vi "Store Configuration Parameters.vi"(8 "error in (no error)":errorcluster, 10 "refnum":T1, 11 "VacuumLines Configuration in":refnum<class "VacuumLines Configuration.lvclass">) -> (0 "error out":errorcluster, 2 "refnum out":T1, 3 "VacuumLines Configuration out":refnum<class "VacuumLines Configuration.lvclass">)   [LabVIEW 2016, in "Hardware.lvlib" / "VacuumLine.lvlib" / "VacuumLines Configuration.lvclass"]
uses:
  <userlib>/Common Components/Hardware/Abstract System/VacuumLine/VacuumLines Configuration/VacuumLines Configuration.lvclass
  <vilib>/Utility/config.llb/Config Data RefNum.ctl
  <userlib>/Common Components/UserPwd DB/UserPwd DB Config/UserPwd DB Configuration.lvclass
  <userlib>/Common Components/Hardware/Abstract System/VacuumLine/VacuumLine Config/VacuumLine Configuration.lvclass
  <vilib>/Utility/config.llb/NI_LVConfig.lvlib
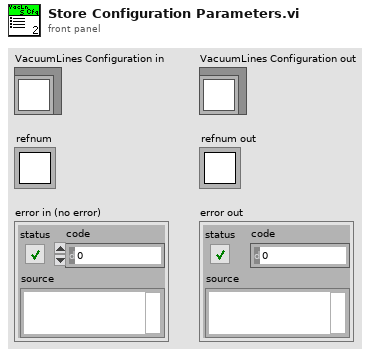
[diagram p1: front panel]
types:
  T1 = typedef "NI_LVConfig.lvlib/Config Data RefNum.ctl" = refnum<k1>
  T2 = cluster{"Conflict Zones":string, "More Valves":string, "Pressure Display":string, "Temperature":string}
  T3 = typedef "Hardware.lvlib/VacuumLine.lvlib/VacuumLines.lvclass/Conflict Zone.ctl" = cluster{"1":cluster{"Label":string, "from":dbl, "to":dbl, "buffer":dbl}, "2":cluster{"Label":string, "from":dbl, "to":dbl, "buffer":dbl}}
  T4 = typedef "Hardware.lvlib/VacuumLine.lvlib/VacuumLines.lvclass/LogicOut.ctl" = cluster{"Label":string, "LogicIO Module":string, "Pin#":u8}
  T5 = typedef "Hardware.lvlib/VacuumLine.lvlib/VacuumLines.lvclass/Gauge Param.ctl" = cluster{"label":string, "Gauge Controller":string, "Channel":enum16{"1", "2", "3", "4", "5", "6", "7", "8"}, "Threshold":dbl}
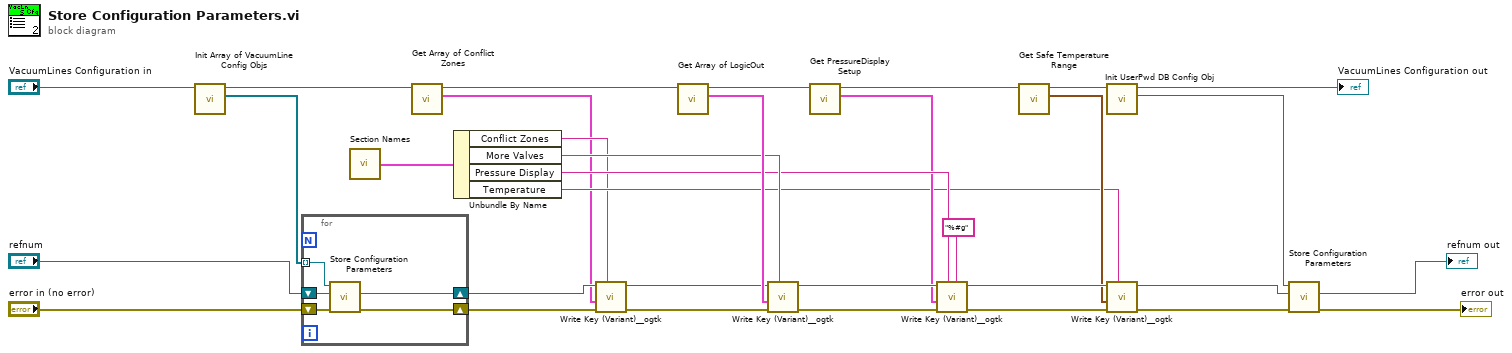
[diagram p0: block diagram]
diagram:
  n1 = call <userlib>:"Init Array of VacuumLine Config Objs.vi"("VacuumLines Configuration in"="VacuumLines Configuration in") -> ("Array of VacuumLine Config Objs"=w28:refnum<class "VacuumLine Configuration.lvclass">[], "VacuumLines Configuration out"=w29:refnum<class "VacuumLines Configuration.lvclass">)  [unwired: 8 in, 1 out]
  n2 = for {
    tunnel: w28 -> [w38] mode=indexing
    shift-right: [w36] -> w7
    shift-left: "refnum" -> [w37]
    shift-right: [w34] -> w30
    shift-left: "error in (no error)" -> [w35]
    n3 = call-dynamic "Store Configuration Parameters.vi"("error in (no error)"=w35, "refnum"=w37, "VacuumLine Configuration in"=w38) -> ("error out"=w34:errorcluster, "refnum out"=w36:T1)  [unwired: 6 in, 1 out]
  }
  n4 = call <userlib>:"Section Names.vi"() -> ("Cluster"=w24:T2)
  n5 = call <userlib>:"Get Array of Conflict Zones.vi"("VacuumLines Configuration in"=w29) -> ("Array of Conflict Zones"=w4:T3[], "VacuumLines Configuration out"=w9:refnum<class "VacuumLines Configuration.lvclass">)  [unwired: 8 in, 1 out]
  n6 = Unbundle By Name(w24) -> ("Conflict Zones"=w5:string, "More Valves"=w23:string, "Pressure Display"=w20:string, "Temperature"=w10:string)
  n7 = call <userlib>:"Write Key (Variant)__ogtk.vi"("section"=w5, "error in (no error)"=w30, "key-value"=w4, "refnum"=w7) -> ("error out"=w8:errorcluster, "refnum out"=w6:T1)  [unwired: 6 in]
  n8 = call <userlib>:"Get Array of LogicOut.vi"("VacuumLines Configuration in"=w9) -> ("Array of LogicOut"=w25:T4[], "VacuumLines Configuration out"=w27:refnum<class "VacuumLines Configuration.lvclass">)  [unwired: 8 in, 1 out]
  n9 = call <userlib>:"Write Key (Variant)__ogtk.vi"("section"=w23, "error in (no error)"=w8, "key-value"=w25, "refnum"=w6) -> ("error out"=w26:errorcluster, "refnum out"=w21:T1)  [unwired: 6 in]
  n10 = call <userlib>:"Get PressureDisplay Setup.vi"("VacuumLines Configuration in"=w27) -> ("PressureDisplay Setup"=w18:T5[], "VacuumLines Configuration out"=w19:refnum<class "VacuumLines Configuration.lvclass">)  [unwired: 8 in, 1 out]
  n11 = call <userlib>:"Write Key (Variant)__ogtk.vi"("float number format"="%#g", "section"=w20, "error in (no error)"=w26, "key-value"=w18, "refnum"=w21) -> ("error out"=w22:errorcluster, "refnum out"=w13:T1)  [unwired: 5 in]
  n12 = call <userlib>:"Get Safe Temperature Range.vi"("VacuumLines Configuration in"=w19) -> ("Safe Temperature Range"=w11:cluster{"min":dbl, "max":dbl}, "VacuumLines Configuration out"=w14:refnum<class "VacuumLines Configuration.lvclass">)  [unwired: 8 in, 1 out]
  n13 = call <userlib>:"Init UserPwd DB Config Obj.vi"("VacuumLines Configuration in"=w14) -> ("UserPwd DB Configuration Obj"=w16:refnum<class "UserPwd DB Configuration.lvclass">, "VacuumLines Configuration out"=→"VacuumLines Configuration out":refnum<class "VacuumLines Configuration.lvclass">)  [unwired: 8 in, 1 out]
  n14 = call <userlib>:"Write Key (Variant)__ogtk.vi"("section"=w10, "error in (no error)"=w22, "key-value"=w11, "refnum"=w13) -> ("error out"=w3:errorcluster, "refnum out"=w12:T1)  [unwired: 6 in]
  n15 = call-dynamic "Store Configuration Parameters.vi"("error in (no error)"=w3, "refnum"=w12, "UserPwd DB Configuration in"=w16) -> ("error out"=→"error out":errorcluster, "refnum out"=→"refnum out":T1)  [unwired: 6 in, 1 out]
